vi "Cubic Deadband Arcade Drive.vi"(9 "YDrive":dbl, 10 "XDrive":dbl, 11 "RobotDriveDevRefIn":T1={"DevStatus"={"status"=FALSE, "code"=0, "source"=""}, "Motors[]"=[], "Square Inputs"=FALSE, "Max Output"=1.0}) -> (3 "RobotDriveDevRef":T1={"DevStatus"={"status"=FALSE, "code"=0, "source"=""}, "Motors[]"=[], "Square Inputs"=FALSE, "Max Output"=1.0})   [LabVIEW 2017]
uses:
  <vilib>/Rock Robotics/WPI/RobotDrive/WPI_RobotDriveDevRef.ctl
  <vilib>/Rock Robotics/WPI/MotorControl/WPI_MotorControlDeviceRef.ctl
  <vilib>/Rock Robotics/WPI/MotorControl/WPI_MotorControlType.ctl
  <vilib>/Rock Robotics/SystemInterfaces/DIO/FPGA_DIOPWMChannel.ctl
  <vilib>/Rock Robotics/WPI/PWM/WPI_PWMDeadband.ctl
  <vilib>/Rock Robotics/SystemInterfaces/DIO/FPGA_DIOChannel.ctl
  <vilib>/Rock Robotics/WPI/RobotDrive/WPI_RobotDriveArcadeDrive_Standard(NoSaturation).vi
panel:
  # "Cubic Arcade Drive\nDeadbands from -0.1 to 0.1"
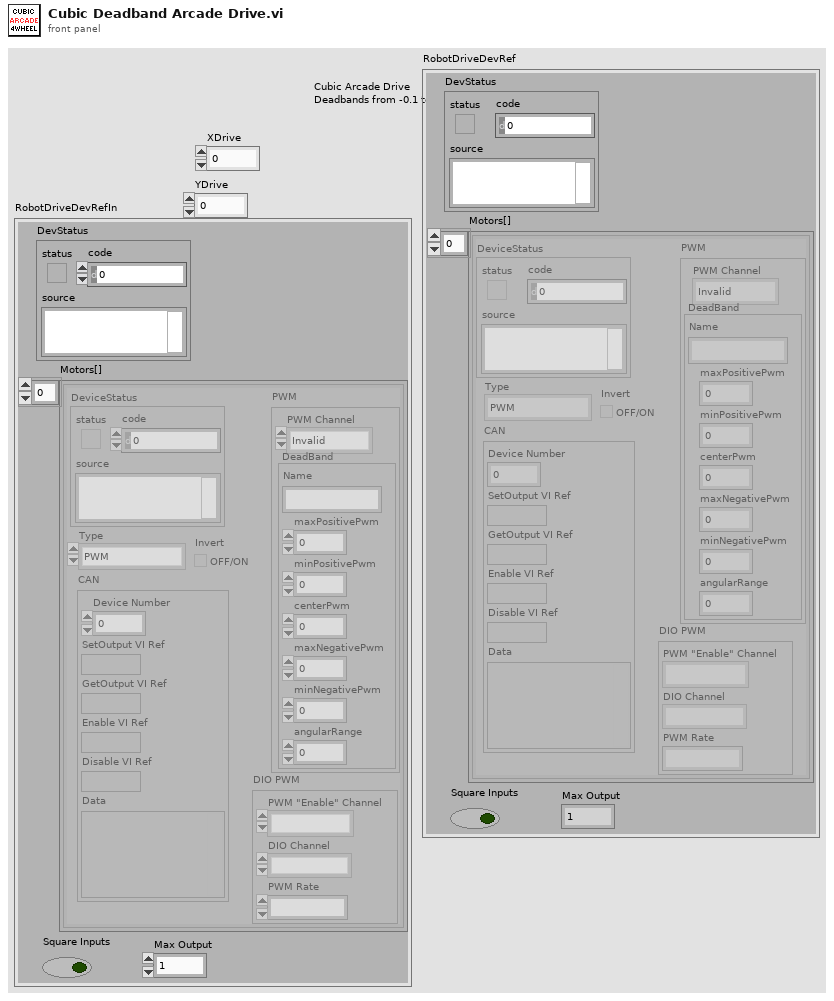
[diagram p1: front panel]
types:
  T1 = typedef "WPI_RobotDriveDevRef.ctl" = cluster{"DevStatus":errorcluster, "Motors[]":T2[], "Square Inputs":bool, "Max Output":dbl}
  T2 = typedef "WPI_MotorControlDeviceRef.ctl" = cluster{"DeviceStatus":errorcluster, "Type":T3, "PWM":cluster{"PWM Channel":T4, "DeadBand":T5}, "CAN":cluster{"Device Number":u8, "SetOutput VI Ref":variant, "GetOutput VI Ref":variant, "Enable VI Ref":variant, "Disable VI Ref":variant, "Data":variant}, "Invert":bool, "DIO PWM":cluster{"PWM \"Enable\" Channel":T4, "DIOChannel":T6, "PWM Rate":dbl}}
  T3 = typedef "WPI_MotorControlType.ctl" = enum16{"PWM", "CAN", "DIO PWM"}
  T4 = typedef "FPGA_DIOPWMChannel.ctl" = enum8{"PWM 0", "PWM 1", "PWM 2", "PWM 3", "PWM 4", "PWM 5", "PWM 6", "PWM 7", "PWM 8", "PWM 9", "PWM MXP 0", "PWM MXP 1", "PWM MXP 2", "PWM MXP 3", "PWM MXP 4", "PWM MXP 5", "PWM MXP 6", "PWM MXP 7", "PWM MXP 8", "PWM MXP 9", "Invalid"}
  T5 = typedef "WPI_PWMDeadband.ctl" = cluster{"Name":string, "maxPositivePwm":i32, "minPositivePwm":i32, "centerPwm":i32, "maxNegativePwm":i32, "minNegativePwm":i32, "angularRange":u16}
  T6 = typedef "FPGA_DIOChannel.ctl" = enum8{"DIO 0", "DIO 1", "DIO 2", "DIO 3", "DIO 4", "DIO 5", "DIO 6", "DIO 7", "DIO 8", "DIO 9", "DIO MXP 0", "DIO MXP 1", "DIO MXP 2", "DIO MXP 3", "DIO MXP 4", "DIO MXP 5", "DIO MXP 6", "DIO MXP 7", "DIO MXP 8", "DIO MXP 9", "DIO MXP 10", "DIO MXP 11", "DIO MXP 12", "DIO MXP 13", "DIO MXP 14", "DIO MXP 15", "SPI Port CS1", "SPI Port CS2", "SPI Port CS3", "SPI Port MISO", "SPI Port MOSI", "Invalid"}
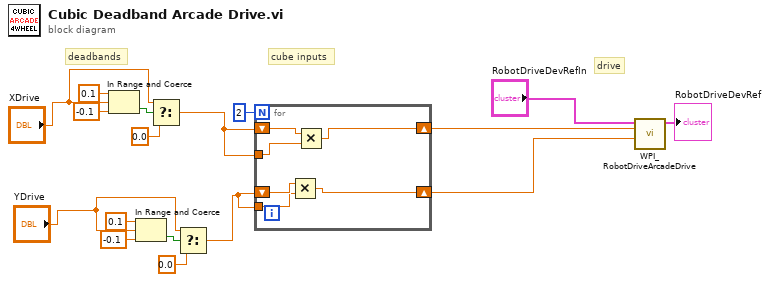
[diagram p0: block diagram]
diagram:
  # "drive"
  # "cube inputs"
  # "deadbands"
  n1 = In Range and Coerce(upper limit=0.1, x="XDrive", lower limit=-0.1) -> (In Range?=w14:bool)  [unwired: 1 out]
  n2 = In Range and Coerce(upper limit=0.1, x="YDrive", lower limit=-0.1) -> (In Range?=w10:bool)  [unwired: 1 out]
  n3 = Select(t="XDrive", s=w14, f=0.0 ("lower limit")) -> (s? t:f=w5:dbl)
  n4 = Select(t="YDrive", s=w10, f=0.0 ("lower limit")) -> (s? t:f=w6:dbl)
  n5 = for {
    N: 2 -> [_]
    shift-right: [w18] -> w3
    shift-left: w6 -> [w20]
    shift-right: [w21] -> w4
    shift-left: w5 -> [w23]
    tunnel: w5 -> [w22]
    tunnel: w6 -> [w19]
    n6 = Multiply(x=w20, y=w19) -> (x*y=w18:dbl)
    n7 = Multiply(x=w23, y=w22) -> (x*y=w21:dbl)
  }
  n8 = call-poly <vilib>:"WPI_RobotDriveArcadeDrive.vi"("Y axis value"=w3, "X axis value"=w4, "RobotDriveDevRef"="RobotDriveDevRefIn") -> ("RobotDriveDevRef"=→"RobotDriveDevRef":T1)  [unwired: 6 in, 2 out]
